vi "Add Standard Claims to Payload.vi"(10 "Additional Standard Claims":T1, 11 "Payload JSON":string) -> (3 "Extended Payload":string)   [LabVIEW 2020, in "JWT.lvlib" / "JWT.lvclass"]
uses:
  JWT.lvclass
  Additional Standard Claims.ctl
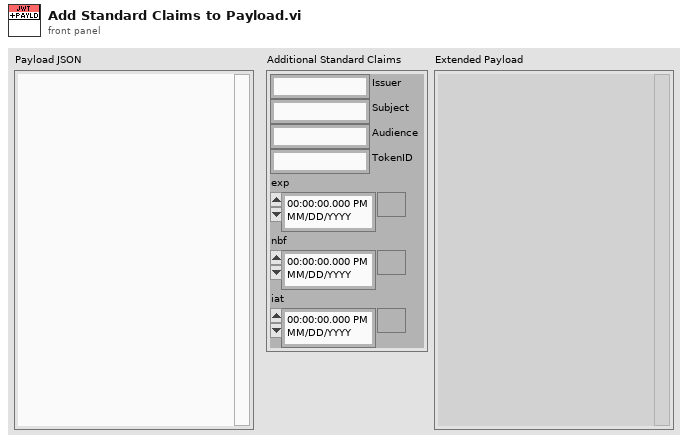
[diagram p1: front panel]
types:
  T1 = typedef "JWT.lvlib/JWT.lvclass/Additional Standard Claims.ctl" = cluster{"Issuer":string, "Subject":string, "Audience":string, "TokenID":string, "exp":timestamp, "nbf":timestamp, "iat":timestamp}
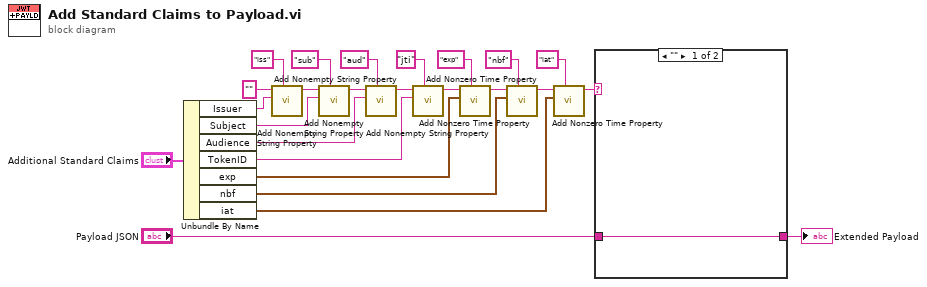
[diagram p0: block diagram]
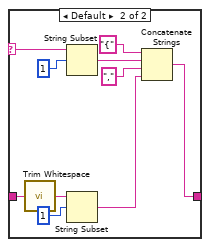
[diagram p2: hidden frame]
diagram:
  n1 = Unbundle By Name("Additional Standard Claims") -> ("Issuer"=w24:string, "Subject"=w22:string, "Audience"=w21:string, "TokenID"=w20:string, "exp"=w10:timestamp, "nbf"=w8:timestamp, "iat"=w6:timestamp)
  n2 = call "Add Nonempty String Property.vi"("Property"="iss", "Value"=w24, "String in"="") -> ("String"=w15:string)  [unwired: 8 in]
  n3 = call "Add Nonempty String Property.vi"("Property"="sub", "Value"=w22, "String in"=w15) -> ("String"=w14:string)  [unwired: 8 in]
  n4 = call "Add Nonempty String Property.vi"("Property"="aud", "Value"=w21, "String in"=w14) -> ("String"=w13:string)  [unwired: 8 in]
  n5 = call "Add Nonempty String Property.vi"("Property"="jti", "Value"=w20, "String in"=w13) -> ("String"=w12:string)  [unwired: 8 in]
  n6 = call "Add Nonzero Time Property.vi"("Property"="exp", "Time Stamp"=w10, "String in"=w12) -> ("String"=w9:string)  [unwired: 8 in]
  n7 = call "Add Nonzero Time Property.vi"("Property"="nbf", "Time Stamp"=w8, "String in"=w9) -> ("String"=w7:string)  [unwired: 8 in]
  n8 = call "Add Nonzero Time Property.vi"("Property"="iat", "Time Stamp"=w6, "String in"=w7) -> ("String"=w3:string)  [unwired: 8 in]
  n9 = case shown="\"\"" w3 {
    selector: w3 -> [_ w36]
    tunnel: [w26 w27] -> w2
    tunnel: "Payload JSON" -> [w26 w32]
    frame "" {
    }
    frame Default {
      n10 = call <vilib>:"Trim Whitespace.vi"("string"=w32) -> ("trimmed string"=w31:string)  [unwired: 1 in]
      n11 = String Subset(string=w36, offset (0)=1) -> (substring=w30:string)  [unwired: 1 in]
      n12 = String Subset(string=w31, offset (0)=1) -> (substring=w28:string)  [unwired: 1 in]
      n13 = Concatenate Strings("{" ("string"), w30, "," ("string"), w28) -> (w27:string)
    }
  }
  "Extended Payload" <- w2
